vi "Keithley Diff Cond.vi"() -> ()   [LabVIEW 2024]
panel:
  in  "Filter Count":u32=10
  in  "Filter":enum16{"Off", "On"}(ring)=enum."On"
  in  "delay [S]":dbl=0.1
  in  "Delta [nA]":dbl=0.25
  in  "Step [nA]":dbl=0.05
  in  "Start [nA]":dbl=10.0
  in  "Range":dbl(ring)=0.01 items=["10 mV"=0.01, "100 mV"=0.1, "1 Volt"=1.0, "10 Volt"=10.0, "100 V"=100.0]
  in  "Average (Sec)":dbl=0.1 min=0.00016667 max=1.0 step=0.00016667 format="%#_2g"
  out "XY Graph":cluster{dbl[], dbl[]}(graph)
  out "Voltage":dbl[](array[numeric])
  out "Resistance":dbl[](array[numeric])
  out "Current":dbl[](array[numeric])
  in  "VISA session":refnum<visa-resource-name>="GPIB0::7::INSTR"
  # "Configure 6221"
  # "Configure 2182 A"
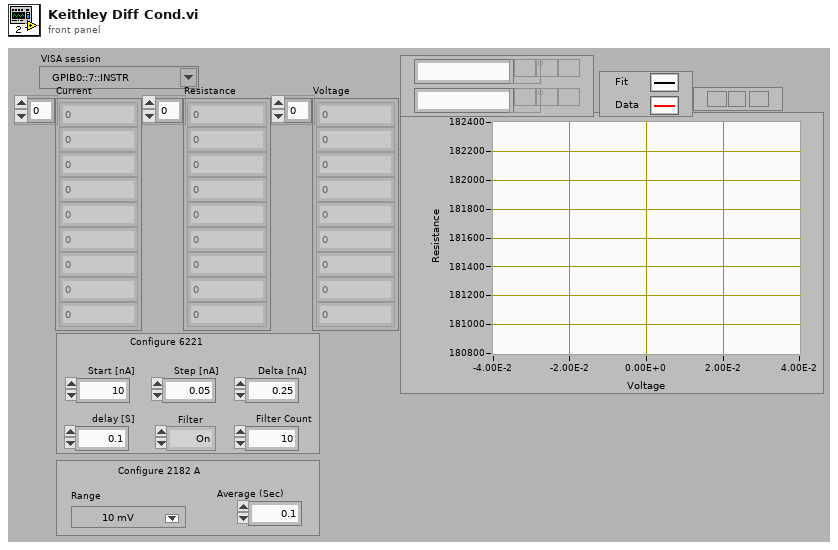
[diagram p1: front panel]
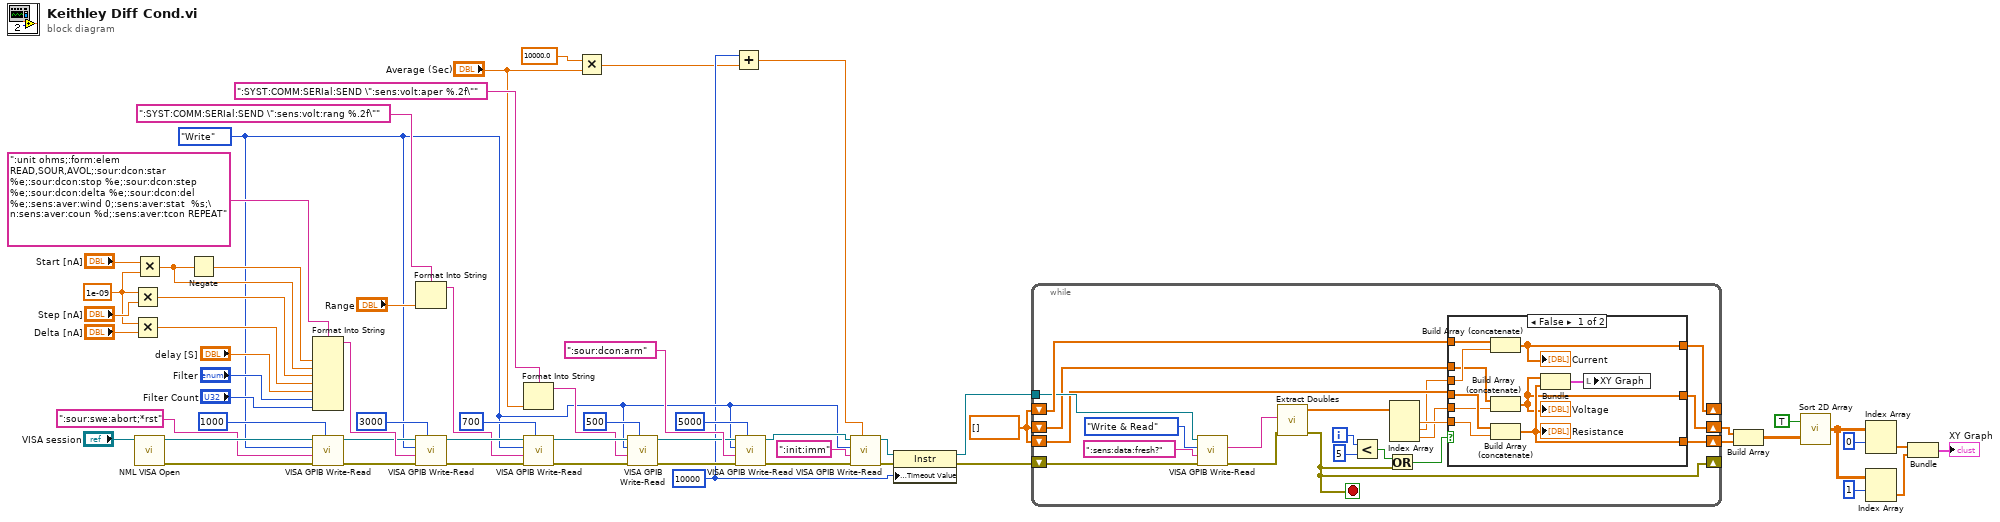
[diagram p0: block diagram]
diagram:
  w7 = enum16{"Write", "Read", "Write & Read"}."Write" ("Action")
  w48 = 1e-09 ("y")
  w3 = u32 10000 ("General Settings:Timeout Value")
  w45 = dbl[] [] ("initialized array")
  n1 = Multiply(x=w48, y="Step [nA]") -> (x*y=w50:dbl)
  n2 = Multiply(x=w48, y="Delta [nA]") -> (x*y=w49:dbl)
  n3 = Multiply(x="Start [nA]", y=w48) -> (x*y=w55:dbl)
  n4 = call "NML VISA Open.vi"("VISA resource name"="VISA session") -> ("error out"=w43:errorcluster, "VISA resource name out"=w44:refnum<visa-resource-name>)  [unwired: 9 in]
  n5 = Negate(x=w55) -> (-x=w56:dbl)
  n6 = Format Into String(format string=":unit ohms;:form:elem READ,SOUR,AVOL;:sour:dcon:star %e;:sour:dcon:stop %e;:sour:dcon:step %e;:sour:dcon:delta %e;:sour:dcon:del %e;:sens:aver:wind 0;:sens:aver:stat  %s;\n:sens:aver:coun %d;:sens:aver:tcon REPEAT" ("String to Write"), w56, w55, w50, w49, "delay [S]", "Filter", "Filter Count") -> (resulting string=w53:string)  [unwired: 2 in, 1 out]
  n7 = call "VISA GPIB Write-Read.vi"("Wait (ms)"=u32 1000 ("milliseconds to wait"), "error in (no error)"=w43, "Command"=":sour:swe:abort;*rst" ("String to Write"), "Action"=w7, "VISA resource name"=w44) -> ("error out"=w8:errorcluster, "dup VISA Session"=w41:refnum<visa-resource-name>)  [unwired: 3 in, 2 out]
  n8 = Format Into String(format string=":SYST:COMM:SERIal:SEND \":sens:volt:rang %.2f\"", "Range") -> (resulting string=w15:string)  [unwired: 2 in, 1 out]
  n9 = call "VISA GPIB Write-Read.vi"("Wait (ms)"=u32 3000 ("milliseconds to wait"), "error in (no error)"=w8, "Command"=w53, "Action"=w7, "VISA resource name"=w41) -> ("error out"=w14:errorcluster, "dup VISA Session"=w18:refnum<visa-resource-name>)  [unwired: 3 in, 2 out]
  n10 = Format Into String(format string=":SYST:COMM:SERIal:SEND \":sens:volt:aper %.2f\"", "Average (Sec)") -> (resulting string=w16:string)  [unwired: 2 in, 1 out]
  n11 = call "VISA GPIB Write-Read.vi"("Wait (ms)"=u32 700 ("wait (mS)"), "error in (no error)"=w14, "Command"=w15, "Action"=w7, "VISA resource name"=w18) -> ("error out"=w13:errorcluster, "dup VISA Session"=w19:refnum<visa-resource-name>)  [unwired: 3 in, 2 out]
  n12 = Multiply(x=10000.0, y="Average (Sec)") -> (x*y=w2:dbl)
  n13 = call "VISA GPIB Write-Read.vi"("Wait (ms)"=u32 500 ("wait (mS)"), "error in (no error)"=w13, "Command"=w16, "Action"=w7, "VISA resource name"=w19) -> ("error out"=w12:errorcluster, "dup VISA Session"=w20:refnum<visa-resource-name>)  [unwired: 3 in, 2 out]
  n14 = Add(x=w3, y=w2) -> (x+y=w4:dbl)
  n15 = call "VISA GPIB Write-Read.vi"("Wait (ms)"=u32 5000 ("milliseconds to wait"), "error in (no error)"=w12, "Command"=":sour:dcon:arm" ("String to Write"), "Action"=w7, "VISA resource name"=w20) -> ("error out"=w24:errorcluster, "dup VISA Session"=w40:refnum<visa-resource-name>)  [unwired: 3 in, 2 out]
  n16 = call "VISA GPIB Write-Read.vi"("Wait (ms)"=w4, "error in (no error)"=w24, "Command"=":init:imm" ("String to Write"), "Action"=w7, "VISA resource name"=w40) -> ("error out"=w25:errorcluster, "dup VISA Session"=w47:refnum<visa-resource-name>)  [unwired: 3 in, 2 out]
  n17 = property class="Instr"(reference=w47, error in=w25, "General Settings:Timeout Value"=w3) -> (reference out=w58:refnum<visa-resource-name>, error out=w59:errorcluster)
  n18 = while {
    shift-right: [w75] -> _
    shift-left: w45 -> [w79]
    shift-right: [w62] -> _
    shift-left: w59 -> [w78]
    tunnel: w58 -> [w77]
    shift-right: [w70] -> w32
    shift-left: w45 -> [w76]
    shift-right: [w69] -> w33
    shift-left: w45 -> [w71]
    i -> [w68]
    stop <- w62 stop-if-true
    n19 = call "VISA GPIB Write-Read.vi"("error in (no error)"=w78, "Command"=":sens:data:fresh?" ("String to Write"), "Action"=enum16{"Write", "Read", "Write & Read"}."Write & Read", "VISA resource name"=w77) -> ("error out"=w61:errorcluster, "String Returned"=w74:string)  [unwired: 4 in, 2 out]
    n20 = call "Extract Doubles.vi"("error in"=w61, "String"=w74) -> ("error out"=w62:errorcluster, "Data"=w73:dbl[])  [unwired: 4 in]
    n21 = Less?(x=w68, y=5) -> (x < y?=w65:bool)
    n22 = Or(x=w65, y=w62) -> (x .or. y?=w66:bool)
    n23 = Index Array(array=w73) -> (element #1=w72:dbl, element #2=w64:dbl, element #3=w63:dbl)  [unwired: 3 in]
    n24 = case shown="False" w66 {
      tunnel: w79 -> [w91 w93]
      tunnel: w76 -> [w90 w94]
      tunnel: [w89 w93] -> w75
      tunnel: w72 -> [w84 _]
      tunnel: w64 -> [w88 _]
      tunnel: w71 -> [w87 w92]
      tunnel: w63 -> [w86 _]
      tunnel: [w85 w94] -> w70
      tunnel: [w83 w92] -> w69
      frame False {
        n25 = Build Array (concatenate)(w91, w88) -> (w89:dbl[])
        "Current" <- w89
        n26 = Build Array (concatenate)(w87, w86) -> (w83:dbl[])
        "Voltage" <- w83
        n27 = Build Array (concatenate)(w90, w84) -> (w85:dbl[])
        "Resistance" <- w85
        n28 = Bundle(w83, w85) -> (w82:cluster{dbl[], dbl[]})  [unwired: 1 in]
        n29 = local write "XY Graph"(w82) -> ()
      }
      frame True {
      }
    }
  }
  n30 = Build Array(w33, w32) -> (w35:dbl[][])
  n31 = call "Sort 2D Array.vi"(1:w35, "First Column"=TRUE) -> (0:w36:dbl[][])
  n32 = Index Array(array=w36, index (row)=0 ("disabled index (col)")) -> (element=w38:dbl[])  [unwired: 1 in]
  n33 = Index Array(array=w36, index (row)=1) -> (element=w37:dbl[])  [unwired: 1 in]
  n34 = Bundle(w38, w37) -> (→"XY Graph":cluster{dbl[], dbl[]})  [unwired: 1 in]
